vi "Avg signal.vi"(0 "Variables in":T2, 2 "Queue in":T1={"Enable zero"=FALSE, "Engr data [Unit]"=[], "Zero button"=FALSE, "Zero [V]"=[], "Timestamp [s]"=0.0, "Write sample"=FALSE, "Record control"=FALSE, "Stop"=FALSE, "error"={"status"=FALSE, "code"=0, "source"=""}, "Raw data [V]\n(all samples)"=[], "Raw data [V]"=[], "Loop count"=1, "Initial time [s]"=0.0, "Scale (0) & Offset (1)"=[], "Image count"=0.0} {"Initial time [s]" format="%_19f"; "Raw data [V]\n(all samples)" format="%0.2f"; "Timestamp [s]" format="%_19f"}) -> (5 "Variables out":T2, 6 "Queue out":T1={"Enable zero"=FALSE, "Engr data [Unit]"=[], "Zero button"=FALSE, "Zero [V]"=[], "Timestamp [s]"=0.0, "Write sample"=FALSE, "Record control"=FALSE, "Stop"=FALSE, "error"={"status"=FALSE, "code"=0, "source"=""}, "Raw data [V]\n(all samples)"=[], "Raw data [V]"=[], "Loop count"=1, "Initial time [s]"=0.0, "Scale (0) & Offset (1)"=[], "Image count"=0.0} {"Initial time [s]" format="%_19f"; "Raw data [V]\n(all samples)" format="%0.2f"; "Timestamp [s]" format="%_19f"}, 7 "Array":dbl[](array[numeric]))   [LabVIEW 2020]
uses:
  <vilib>/Analysis/NI_AALBase.lvlib
  <vilib>/Analysis/baseanly.llb/Mean (DBL).vi
  Constants.ctl
  Queue.ctl
panel:
  # "Description: \nAdds zero value to raw data when enabled. \nCaptures raw data as new zero value when zero button is pressed."
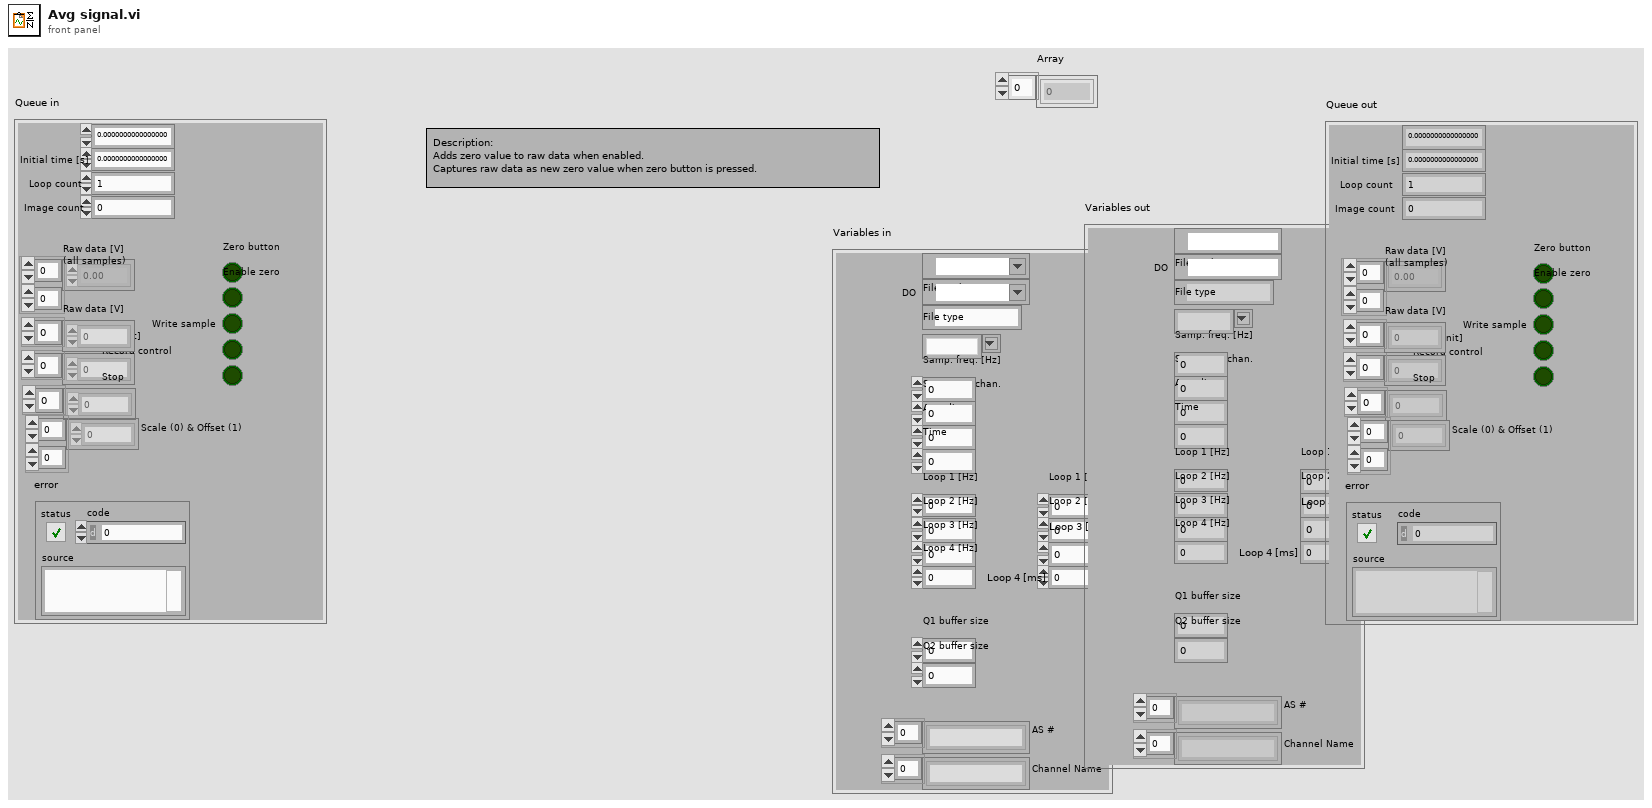
[diagram p1: front panel]
types:
  T1 = typedef "Queue.ctl" = cluster{"Enable zero":bool, "Engr data [Unit]":dbl[], "Zero button":bool, "Zero [V]":dbl[], "Timestamp [s]":dbl, "Write sample":bool, "Record control":bool, "Stop":bool, "error":errorcluster, "Raw data [V]\n(all samples)":dbl[][], "Raw data [V]":dbl[], "Loop count":i64, "Initial time [s]":dbl, "Scale (0) & Offset (1)":dbl[][], "Image count":dbl}
  T2 = typedef "Constants.ctl" = cluster{"Time":u16, "Samp. freq. [Hz]":dbl, "Samp. per chan.":i32, "Avg. div.":i32, "File path":path, "AI":refnum<k21>, "Loop 1 [Hz]":dbl, "Loop 2 [Hz]":dbl, "Loop 3 [Hz]":dbl, "Loop 1 [ms]":dbl, "Loop 2 [ms]":dbl, "Loop 3 [ms]":dbl, "Q1 buffer size":i32, "Q2 buffer size":i32, "File type":string, "Loop 4 [Hz]":dbl, "Loop 4 [ms]":dbl, "Channel Name":string[], "AS #":string[], "DO":refnum<k21>}
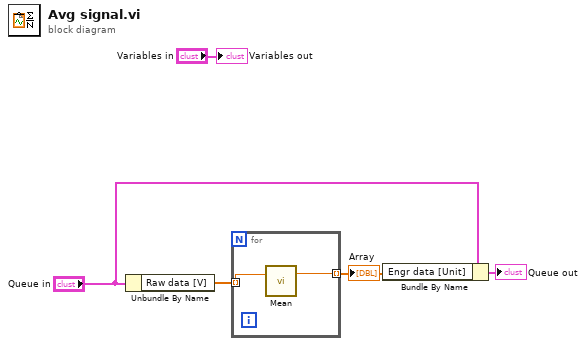
[diagram p0: block diagram]
diagram:
  n1 = Unbundle By Name("Queue in") -> ("Raw data [V]"=w4:dbl[])
  n2 = for {
    tunnel: w4 -> [w7] mode=indexing
    tunnel: [w6] -> w1 mode=indexing
    n3 = call-poly <vilib>:"Mean.vi"("X"=w7) -> ("mean"=w6:dbl)  [unwired: 1 out]
  }
  "Array" <- w1
  n4 = Bundle By Name(cluster="Queue in", "Engr data [Unit]"=w1) -> (→"Queue out":T1)
  "Variables out" <- "Variables in"
